vi "PH_TKTDS-30xx.check Error.vi"(0 "i ref in":refnum<vi>, 2 "Waiting Time [ms]":u32, 5 "error in":errorcluster) -> (14 "i ref out":refnum<vi>, 19 "error out":errorcluster)   [LabVIEW 2014, in "PH_TKTDS-30xx.lvlib"]
doc: "This VI has to be set after any communication with the hardware: It queries the hardware error and sets the busy flag depending on the result to false or failure; the hardware error is indicated at the GUI elemnt (tip strip). It is the counterpart to \"start communication\"."
uses:
  PH_TKTDS-30xx.lvlib
  PH_Basics/PH_StatusHandler/PH_StatusHandler.Status.ctl
  PH_Basics/PH_StatusHandler/PH_StatusHandler.lvlib
  instr.lib/TKDS3032-PHELIX/tktds3032-PHELIX - Driver np.lvlib
  PH_Basics/PH_Common/PH_Common.lvlib
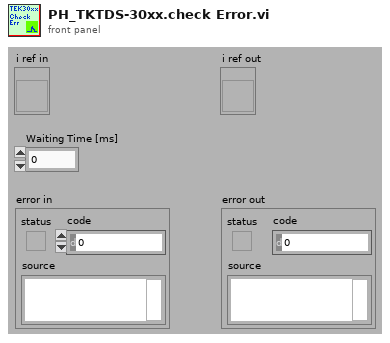
[diagram p1: front panel]
types:
  T1 = typedef "PH_TKTDS-30xx.lvlib/PH_TKTDS-30xx.i attribute.ctl" = cluster{"Default VISA Resource":string, "VISA Resource Name":refnum<visa-resource-name>, "Revision":cluster{"Instrument Driver":string, "Instrument Firmware":string}, "Selftest":cluster{"Result":u32, "Message":string}, "Channels":T2[], "Trigger Configuration":T4, "Acquisition Configuration":T5, "Fetched Waveforms":T6[], "GUI Refs":T7, "State":T8, "Error Message":string, "Allow Prdc Loop?":bool}
  T2 = typedef "PH_TKTDS-30xx.lvlib/PH_TKTDS-30xx.Channel Config.ctl" = cluster{"Channel Name":string, "Input Impedance":string, "Max Input Frequency":string, "Vertical Coupling":i32, "Channel Enabled":bool, "Probe Attenuation":dbl, "Vertical Range":dbl, "Vertical Offset":dbl, "Waveform Limits":T3}
  T3 = typedef "PH_TKTDS-30xx.lvlib/PH_TKTDS-30xx.Waveform Limits.ctl" = cluster{"Start":i32, "End":i32}
  T4 = typedef "PH_TKTDS-30xx.lvlib/PH_TKTDS-30xx.Trigger Config.ctl" = cluster{"Source":string, "Slope":i32, "Level [V]":dbl}
  T5 = typedef "PH_TKTDS-30xx.lvlib/PH_TKTDS-30xx.Acquisition Config.ctl" = cluster{"Time base":dbl, "Record Length":u16, "Start Time":dbl, "Type":i32, "Continuous":bool}
  T6 = typedef "PH_TKTDS-30xx.lvlib/PH_TKTDS-30xx.fetched Waveform.ctl" = cluster{"Source":string, "Actual Points":u32, "Initial X":dbl, "X Increment":dbl, "Waveform Array":dbl[]}
  T7 = typedef "PH_TKTDS-30xx.lvlib/PH_TKTDS-30xx.GUI Refs.ctl" = cluster{"Trigger":refnum<vi>, "Acquisition":refnum<vi>, "State":refnum<vi>, "Delete":refnum<vi>, "Channel to be positioned":refnum<vi>, "Postion":refnum<vi>, "Display Intensity":refnum<vi>, "VISA Resource":refnum<vi>, "Channels":refnum<vi>[], "Graphs":refnum<vi>[]}
  T8 = typedef "PH_StatusHandler.lvlib/PH_StatusHandler.Status.ctl" = i16
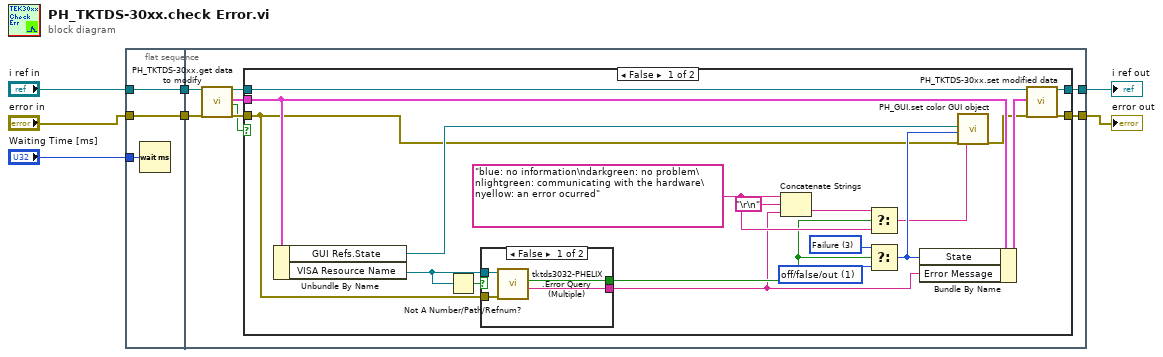
[diagram p0: block diagram]
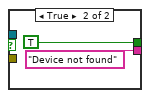
[diagram p2: hidden frame]
diagram:
  n1 = flat-sequence {
    tunnel: "i ref in" -> [w9]
    tunnel: "error in" -> [w10]
    tunnel: [w10] -> w3
    tunnel: [w9] -> w2
    tunnel: "Waiting Time [ms]" -> [w8]
    tunnel: [w15] -> w7
    tunnel: [w13] -> w5
    tunnel: w3 -> [w14]
    tunnel: w2 -> [w12]
    frame #0 {
      n2 = Wait (ms)(milliseconds to wait=w8) -> ()  [unwired: 1 out]
    }
    frame #1 {
      n3 = call "PH_TKTDS-30xx.get data to modify.vi"("i ref in"=w12, "error in (no error)"=w14) -> ("i ref out"=w16:refnum<vi>, "i attribute"=w18:T1, "timed out"=w11:bool, "error out"=w17:errorcluster)  [unwired: 14 in]
      n4 = case shown="False" w11 {
        tunnel: [w37 w44] -> w15
        tunnel: w17 -> [w21 w44]
        tunnel: w16 -> [w36 w45]
        tunnel: [w35 w45] -> w13
        tunnel: w18 -> [w33 _]
        frame False {
          w25 = "blue: no information\ndarkgreen: no problem\nlightgreen: communicating with the hardware\nyellow: an error ocurred"
          w31 = T8 1 items=["no info", "off/false/out", "on/true/in", "Failure", "Alarm", "Status 1", "Status 2", "Status 3"] ("f")
          w32 = T8 3 items=["no info", "off/false/out", "on/true/in", "Failure", "Alarm", "Status 1", "Status 2", "Status 3"] ("State")
          n5 = Unbundle By Name(w33) -> ("GUI Refs.State"=w29:refnum<vi>, "VISA Resource Name"=w20:refnum<visa-resource-name>)
          n6 = Not A Number/Path/Refnum?(number/path/refnum=w20) -> (NaN/Path/Refnum?=w19:bool)
          n7 = case shown="False" w19 {
            tunnel: [w41 TRUE ("error")] -> w23
            tunnel: [w40 "Device not found" ("error message")] -> w22
            tunnel: w21 -> [w39 _]
            tunnel: w20 -> [w38 _]
            frame False {
              n8 = call "tktds3032-PHELIX.Error Query (Multiple).vi"("error in (no error)"=w39, "VISA Resource Name"=w38) -> ("error message"=w40:string, "error"=w41:bool)  [unwired: 6 in, 2 out]
            }
            frame True {
            }
          }
          n9 = Concatenate Strings(w25, "\r\n", w22) -> (w24:string)
          n10 = Select(t=w24, s=w23, f=w25) -> (s? t:f=w27:string)
          n11 = Select(t=w32, s=w23, f=w31) -> (s? t:f=w28:T8)
          n12 = Bundle By Name(cluster=w33, "State"=w28, "Error Message"=w22) -> (w34:T1)
          n13 = call "PH_GUI.set color GUI object.vi"("GUI object Ref"=w29, "State"=w28, "error in (no error)"=w21, "Tip Strip (N/A)"=w27) -> ("error out"=w30:errorcluster)  [unwired: 15 in]
          n14 = call "PH_TKTDS-30xx.set modified data.vi"("i ref in"=w36, "i attribute"=w34, "error in (no error)"=w30) -> ("i ref out"=w35:refnum<vi>, "error out"=w37:errorcluster)  [unwired: 15 in]
        }
        frame True {
        }
      }
    }
  }
  "error out" <- w7
  "i ref out" <- w5
